vi "sio read.vi"(9 "len":i32, 10 "buf":string, 11 "port":i32) -> (2 "buf out":string, 3 "function return":i32)   [LabVIEW 2012, in "PCOMM.lvlib"]
doc: "int WINAPI sio_read(int port, char *buf, int len);"
uses:
  PCOMM.lvlib
  #001 2018-09-10/Data/PCOMM.DLL
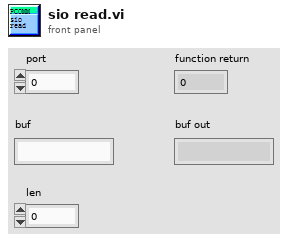
[diagram p1: front panel]
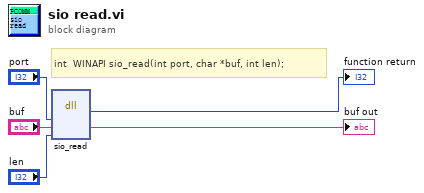
[diagram p0: block diagram]
diagram:
  # "int  WINAPI sio_read(int port, char *buf, int len);"
  n1 = dll-call lib="E:/ProJect/#008 ESDMonitor/#002 Labview/#001 2018-09-10/Data/PCOMM.DLL" fn="sio_read"("port"="port", "buf"="buf", "len"="len") -> ("返回类型"=→"function return":i32, "buf"=→"buf out":string)  [unwired: 5 in, 2 out]
